vi "APC_9049_HRL_MAPO.vi"(3 "IIR Filter Cluster":T1, 4 "Pcyl":dbl[](array[numeric])) -> (0 "PcylHPfilt":dbl[](array[numeric]), 1 "MAPO":dbl)   [LabVIEW 2020]
panel:
  in  "knock window length [sample]":i32=1500
  in  "knock window position [sample]":i32=3000
  in  "Graph":bool
  out "Pressure filtering":dbl[][](graph)
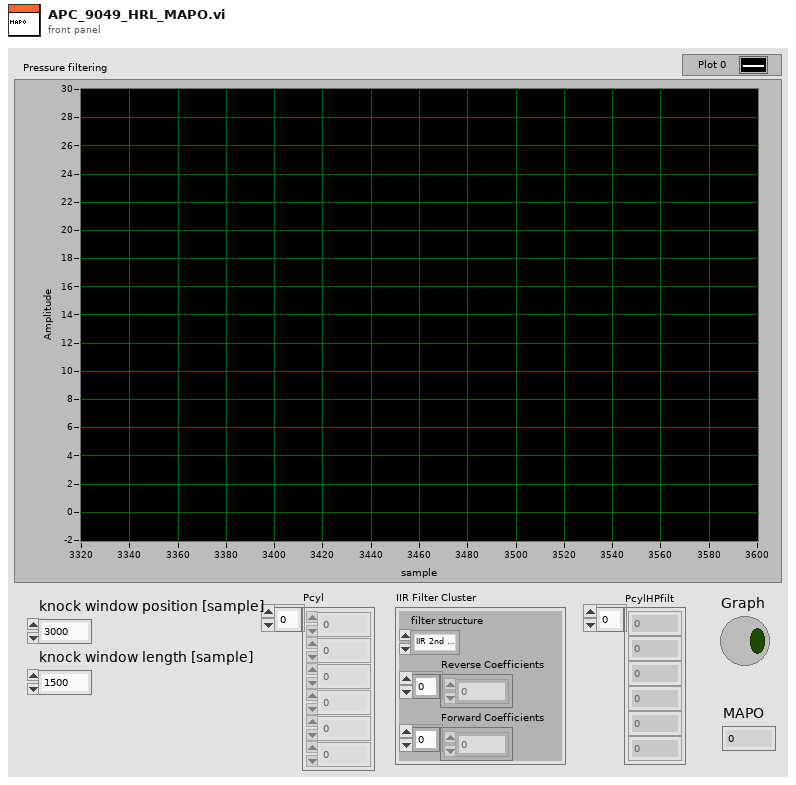
[diagram p1: front panel]
types:
  T1 = cluster{"filter structure":enum32{"IIR 2nd Order", "IIR 4th Order"}, "Reverse Coefficients":dbl[], "Forward Coefficients":dbl[]}
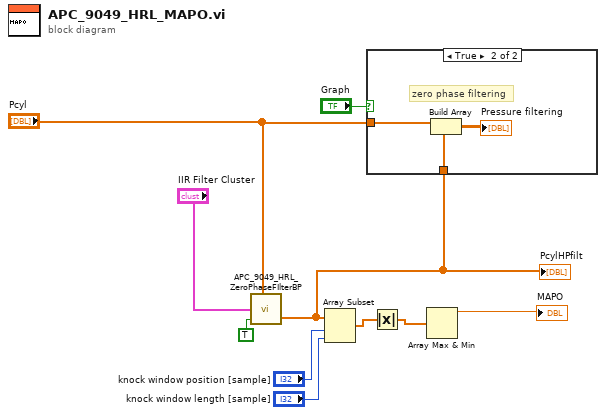
[diagram p0: block diagram]
diagram:
  n1 = call "APC_9049_HRL_ZeroPhaseFIlterBP.vi"("Init value removal"=TRUE ("Init value compensation"), "IIR Filter Cluster"="IIR Filter Cluster", "Pcyl"="Pcyl") -> ("Pcylfilt"=w4:dbl[])  [unwired: 1 out]
  "PcylHPfilt" <- w4
  n2 = Array Subset(array=w4, index="knock window position [sample]", length="knock window length [sample]") -> (w8:dbl[])
  n3 = case shown="True" "Graph" {
    tunnel: "Pcyl" -> [_ w13]
    tunnel: w4 -> [_ w11]
    frame False {
    }
    frame True {
      # "zero phase filtering"
      n4 = Build Array(w13, w11) -> (→"Pressure filtering":dbl[][])
    }
  }
  n5 = Absolute Value(x=w8) -> (abs(x)=w7:dbl[])
  n6 = Array Max & Min(array=w7) -> (max value=→"MAPO":dbl)  [unwired: 3 out]
